vi "PIM Base Order to IM Order.vi"(1 "Base Order (0)":u8) -> (4 "IM Order":u8, 5 "IM Order String":string)   [LabVIEW 2011]
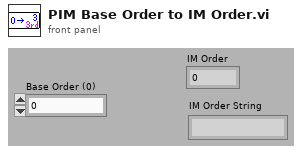
[diagram p1: front panel]
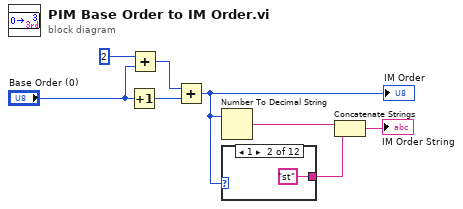
[diagram p0: block diagram]
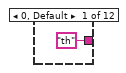
[diagram p2: hidden frame]
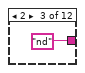
[diagram p3: hidden frame]
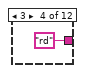
[diagram p4: hidden frame]
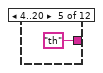
[diagram p5: hidden frame]
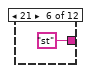
[diagram p6: hidden frame]
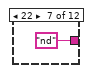
[diagram p7: hidden frame]
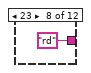
[diagram p8: hidden frame]
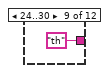
[diagram p9: hidden frame]
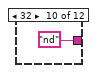
[diagram p10: hidden frame]
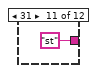
[diagram p11: hidden frame]
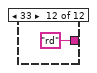
[diagram p12: hidden frame]
diagram:
  n1 = Increment(x="Base Order (0)") -> (x+1=w5:u8)
  n2 = Add(x=u8 2, y="Base Order (0)") -> (x+y=w6:u8)
  n3 = Add(x=w6, y=w5) -> (x+y=w1:u8)
  "IM Order" <- w1
  n4 = Number To Decimal String(number=w1) -> (decimal integer string=w3:string)  [unwired: 1 out]
  n5 = case shown="1" w1 {
    tunnel: ["th" "st" "nd" "rd" "th" "st" "nd" "rd" "th" "nd" "st" "rd"] -> w4
    frame 0, Default {
    }
    frame 1 {
    }
    frame 2 {
    }
    frame 3 {
    }
    frame 4..20 {
    }
    frame 21 {
    }
    frame 22 {
    }
    frame 23 {
    }
    frame 24..30 {
    }
    frame 32 {
    }
    frame 31 {
    }
    frame 33 {
    }
  }
  n6 = Concatenate Strings(w3, w4) -> (→"IM Order String":string)
